vi "gfitsio-check-col-for-write.vi"(4 "units":string, 5 "cfitsio datatype":T1=82 items=["ANY_HDU"=-1, "IMAGE_HDU"=0, "ASCII_TBL"=1, "BINARY_TBL"=2], 6 "row":i32, 7 "column":string, 8 "error in (no error)":errorcluster, 9 "size (-1:variable)":i32=-1, 11 "gfits refnum":T2=refnum) -> (0 "error out":errorcluster, 2 "colnum":i32, 3 "dup gfits refnum":T2)   [LabVIEW 2011, in "gfitsio.lvlib"]
uses:
  gfitsio.lvlib
  gfitsio-refnum.ctl
  cfitsio-hdutypes.ctl
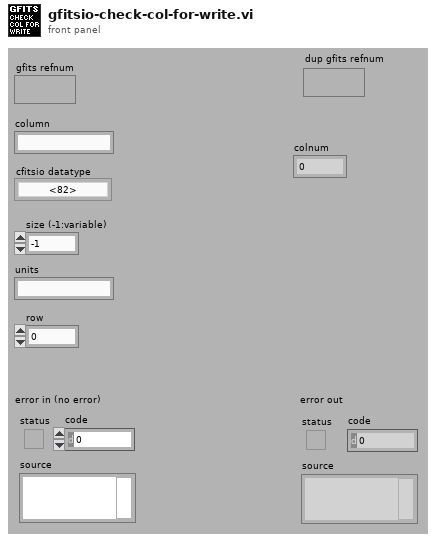
[diagram p1: front panel]
types:
  T1 = typedef "gfitsio.lvlib/cfitsio-hdutypes.ctl" = i32
  T2 = typedef "gfitsio.lvlib/gfitsio-refnum.ctl" = refnum<k1>
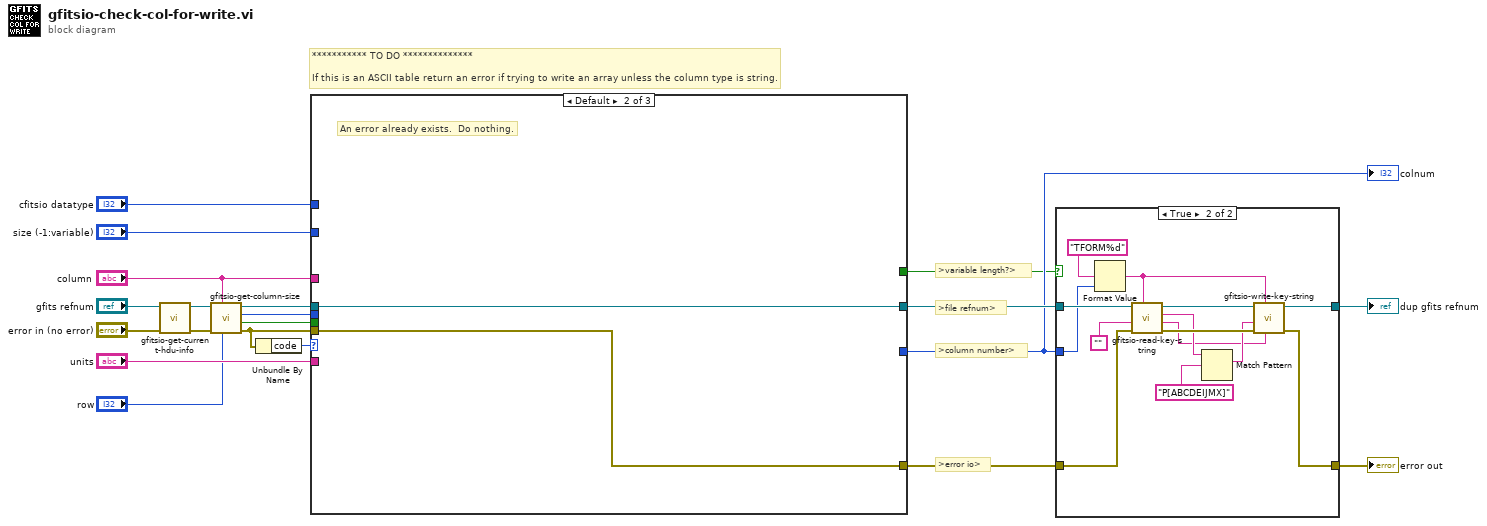
[diagram p0: block diagram]
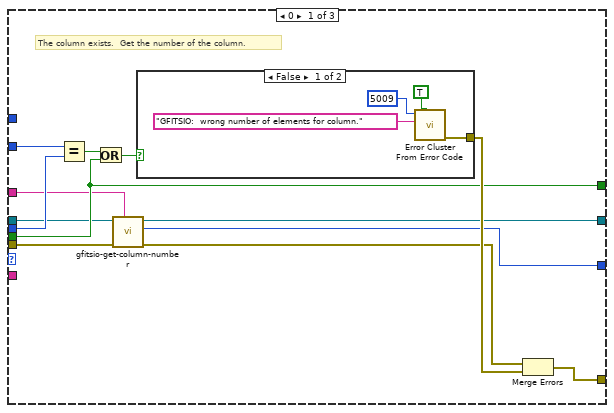
[diagram p2: hidden frame]
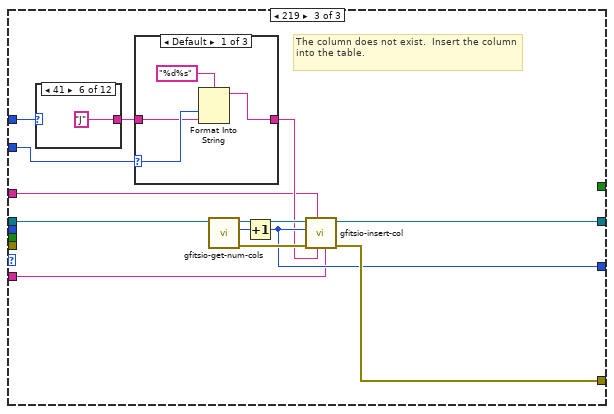
[diagram p4: hidden frame]
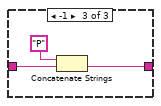
[diagram p6: hidden frame]
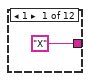
[diagram p7: hidden frame]
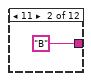
[diagram p8: hidden frame]
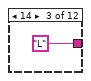
[diagram p9: hidden frame]
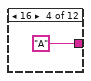
[diagram p10: hidden frame]
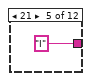
[diagram p11: hidden frame]
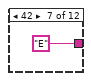
[diagram p12: hidden frame]
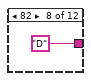
[diagram p13: hidden frame]
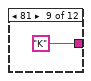
[diagram p14: hidden frame]
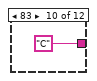
[diagram p15: hidden frame]
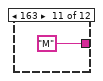
[diagram p16: hidden frame]
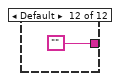
[diagram p17: hidden frame]
diagram:
  # ">error io>"
  # ">file refnum>"
  # ">column number>"
  # ">variable length?>"
  # "*********** TO DO **************\n\nIf this is an ASCII table return an error if trying to write an array unless the column type is string."
  n1 = call "gfitsio-get-current-hdu-info.vi"("error in (no error)"="error in (no error)", "gfits refnum"="gfits refnum") -> ("error out"=w3:errorcluster, "dup gfits refnum"=w4:T2)  [unwired: 5 in, 3 out]
  n2 = call "gfitsio-get-column-size.vi"("row"="row", "column"="column", "error in (no error)"=w3, "gfits refnum"=w4) -> ("error out"=w9:errorcluster, "variable length?"=w2:bool, "nelements"=w7:i32, "dup gfits refnum"=w8:T2)  [unwired: 4 in]
  n3 = Unbundle By Name(w9) -> ("code"=w10:i32)
  n4 = case shown="Default" w10 {
    tunnel: w9 -> [w26 w39 _]
    tunnel: [w29 w39 w52] -> w15
    tunnel: [w23 w38 w51] -> w14
    tunnel: w8 -> [w25 w38 w48]
    tunnel: [w21 _ w46] -> w12
    tunnel: "units" -> [_ _ w41]
    tunnel: w7 -> [w28 _ _]
    tunnel: "size (-1:variable)" -> [w33 _ w43]
    tunnel: "cfitsio datatype" -> [_ _ w45]
    tunnel: [w27 _ _] -> w11
    tunnel: "column" -> [w24 _ w40]
    tunnel: w2 -> [w27 _ _]
    frame 0 {
      # "The column exists.  Get the number of the column."
      n5 = Equal?(x=w33, y=w28) -> (x = y?=w32:bool)
      n6 = Or(x=w32, y=w27) -> (x .or. y?=w31:bool)
      n7 = call "gfitsio-get-column-number.vi"("column"=w24, "error in (no error)"=w26, "gfits refnum"=w25) -> ("error out"=w22:errorcluster, "colnum"=w21:i32, "dup gfits refnum"=w23:T2)  [unwired: 6 in]
      n8 = case shown="False" w31 {
        tunnel: [w35 _] -> w30
        frame False {
          n9 = call <vilib>:"Error Cluster From Error Code.vi"("show call chain? (False)"=TRUE, "error message (\"\")"="GFITSIO:  wrong number of elements for column." ("error message (\"\")"), "error code (0)"=5009) -> ("error out"=w35:errorcluster)  [unwired: 6 in]
        }
        frame True {
        }
      }
      n10 = Merge Errors(w22, w30) -> (w29:errorcluster)
    }
    frame Default {
      # "An error already exists.  Do nothing."
    }
    frame 219 {
      # "The column does not exist.  Insert the column into the table."
      n11 = case shown="41" w45 {
        tunnel: ["X" "B" "L" "A" "I" "J" "E" "D" "K" "C" "M" ""] -> w44
        frame 1 {
        }
        frame 11 {
        }
        frame 14 {
        }
        frame 16 {
        }
        frame 21 {
        }
        frame 41 {
        }
        frame 42 {
        }
        frame 82 {
        }
        frame 81 {
        }
        frame 83 {
        }
        frame 163 {
        }
        frame Default {
        }
      }
      n12 = case shown="Default" w43 {
        selector: w43 -> [w56 _ _]
        tunnel: w44 -> [w55 w57 w60]
        tunnel: [w54 w57 w58] -> w42
        frame Default {
          n13 = Format Into String(format string="%d%s" ("initial string"), w56, w55) -> (resulting string=w54:string)  [unwired: 2 in, 1 out]
        }
        frame 1 {
        }
        frame -1 {
          n14 = Concatenate Strings("P" ("string"), w60) -> (w58:string)
        }
      }
      n15 = call "gfitsio-get-num-cols.vi"("gfits refnum"=w48) -> ("error out"=w50:errorcluster, "number of columns"=w49:i32, "dup gfits refnum"=w47:T2)  [unwired: 8 in]
      n16 = Increment(x=w49) -> (x+1=w46:i32)
      n17 = call "gfitsio-insert-col.vi"("tunits"=w41, "tform"=w42, "ttype"=w40, "error in (no error)"=w50, "insertion point (0:1st column)"=w46, "gfits refnum"=w47) -> ("error out"=w52:errorcluster, "dup gfits refnum"=w51:T2)  [unwired: 4 in]
    }
  }
  "colnum" <- w12
  n18 = case shown="True" w11 {
    tunnel: [w73 w88] -> w16
    tunnel: w15 -> [w73 w85]
    tunnel: w14 -> [w74 w84]
    tunnel: [w74 w83] -> w13
    tunnel: w12 -> [_ w79]
    frame False {
    }
    frame True {
      n19 = Format Value(format string="TFORM%d", value (0)=w79) -> (output string=w76:string)  [unwired: 1 in]
      n20 = call "gfitsio-read-key-string.vi"("keyname"=w76, "error in (no error)"=w85, "default value"="", "gfits refnum"=w84) -> ("error out"=w86:errorcluster, "comment"=w75:string, "value"=w78:string, "dup gfits refnum"=w87:T2)  [unwired: 4 in]
      n21 = Match Pattern(string=w78, regular expression="P[ABCDEIJMX]") -> (match substring=w77:string)  [unwired: 1 in, 3 out]
      n22 = call "gfitsio-write-key-string.vi"("comment"=w75, "keyname"=w76, "error in (no error)"=w86, "value"=w77, "gfits refnum"=w87) -> ("error out"=w88:errorcluster, "dup gfits refnum"=w83:T2)  [unwired: 5 in]
    }
  }
  "error out" <- w16
  "dup gfits refnum" <- w13
